vi "Read ChannelData.vi"(8 "error in (no error)":errorcluster, 11 "EMG in":refnum<class "EMG.lvclass">) -> (0 "error out":errorcluster, 2 "ChannelData":dbl[][](array[numeric]), 3 "EMG out":refnum<class "EMG.lvclass">)   [LabVIEW 2015, in "EMG.lvclass"]
uses:
  EMG.lvclass
  EMG.lvclass/EMG.ctl
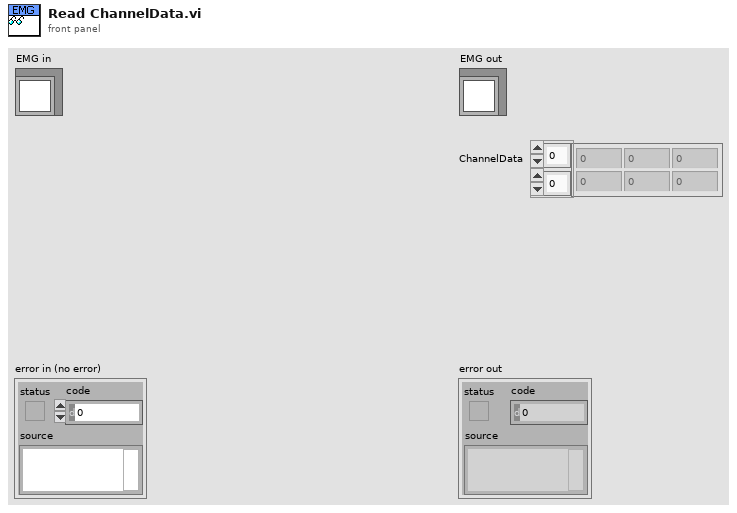
[diagram p1: front panel]
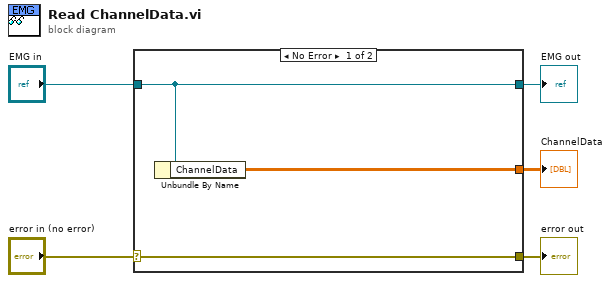
[diagram p0: block diagram]
diagram:
  n1 = case shown="No Error" "error in (no error)" {
    selector: "error in (no error)" -> [w8 w9]
    tunnel: [w8 w9] -> w4
    tunnel: [w7 w10] -> w2
    tunnel: "EMG in" -> [w7 w10]
    tunnel: [w6 _] -> w1
    frame No Error {
      n2 = Unbundle By Name(w7) -> ("ChannelData"=w6:dbl[][])
    }
    frame Error {
    }
  }
  "error out" <- w4
  "EMG out" <- w2
  "ChannelData" <- w1
